vi "dashboard_motors_calibration.vi"() -> ()   [LabVIEW 2022 SP3]
panel:
  out "Applied R PWM":dbl
  in  "Tau u (s)":dbl min=0.0 max=30.0 step=0.01 format="%.2g"
  out "Applied L PWM":dbl
  in  "Stop":bool
  out "Write Count":i32
  out "Read Count":i32
  in  "Reset Communication":bool
  in  "USB Port":refnum<visa-resource-name>
  out "u":dbl format="%.2g"
  out "D":dbl format="%.2g"
  out "I":dbl format="%.2g"
  out "P":dbl format="%.2g"
  in  "Tau D (s)":dbl min=0.0 max=30.0 step=0.01 format="%.2g"
  in  "Td":dbl min=0.0 max=50.0 step=0.01 format="%.2g"
  in  "Ti":dbl=100.0 min=0.0 max=100.0 step=0.01 format="%.2g"
  in  "Kc":dbl min=0.0 max=50.0 step=0.01 format="%.2g"
  out "Flag AntiWindUp":bool
  out "Error (°)":dbl
  out "Controller":cluster{" P":dbl, "I":dbl, "D":dbl, "u":dbl}(graph)
  out "Error":cluster{" error":dbl, "Filtered_error":dbl}(graph)
  in  "PWM %":dbl(slide) min=-100.0 max=100.0 step=1.0 scale=-100.0..100.0
  in  "Setpoint (RPM)":dbl(slide) min=-1500.0 max=1500.0 step=100.0 scale=-1500.0..1500.0
  in  "Manual Control":bool=TRUE
  out "Left Motor":T1(graph)
  out "Right Motor":T2(graph)
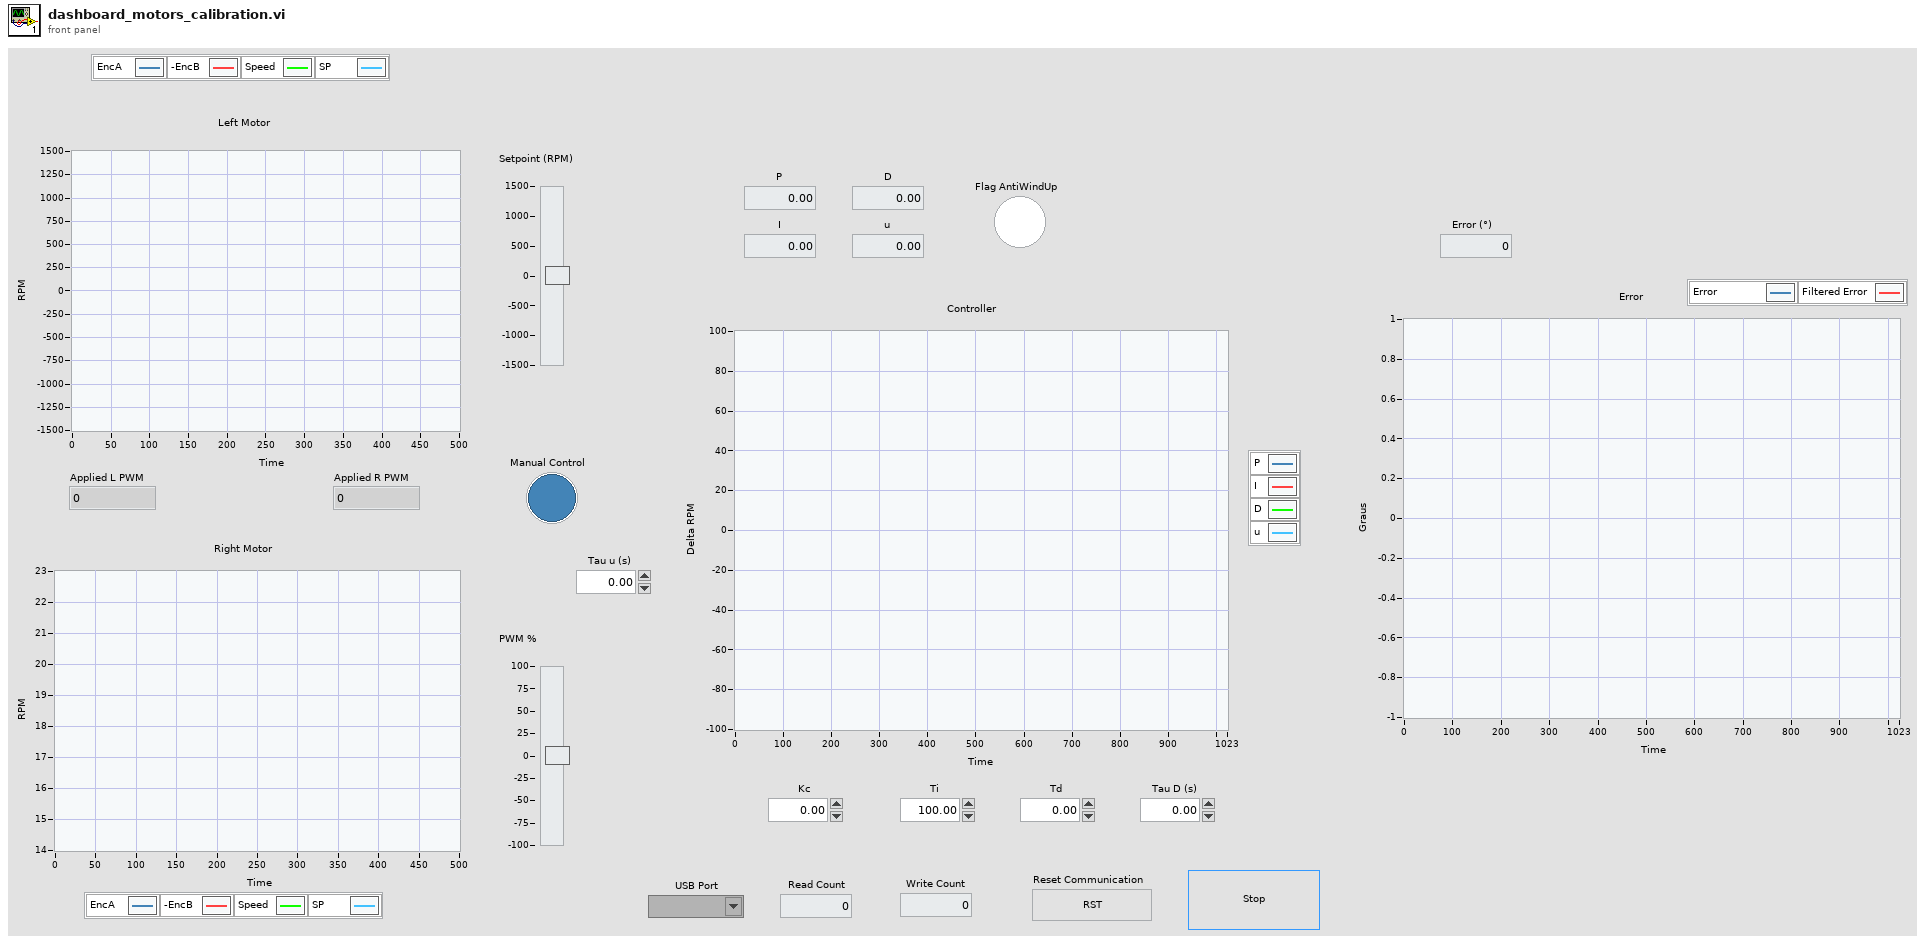
[diagram p1: front panel]
types:
  T1 = cluster{"l_sp":dbl, "l_speed":dbl, dbl, "Setpoint (RPM)":dbl}
  T2 = cluster{"r_sp":dbl, " r_speed":dbl, dbl, "Setpoint (RPM)":dbl}
  T3 = cluster{"Manual Control":bool, bool, "Setpoint (RPM)":dbl, "PWM %":dbl, "Tau u (s)":dbl, "Kc":dbl, "Ti":dbl, "Td":dbl, "Tau D (s)":dbl, dbl, dbl, dbl, dbl, dbl, dbl, dbl}
  T4 = cluster{"l_sp":dbl, "l_speed":dbl, "r_sp":dbl, " r_speed":dbl, " error":dbl, "Filtered_error":dbl, " P":dbl, "I":dbl, "D":dbl, "u":dbl, "sat_flag":bool, " IR":bool[], "A_":dbl, " B_":dbl, " C_":dbl, "D_":dbl}
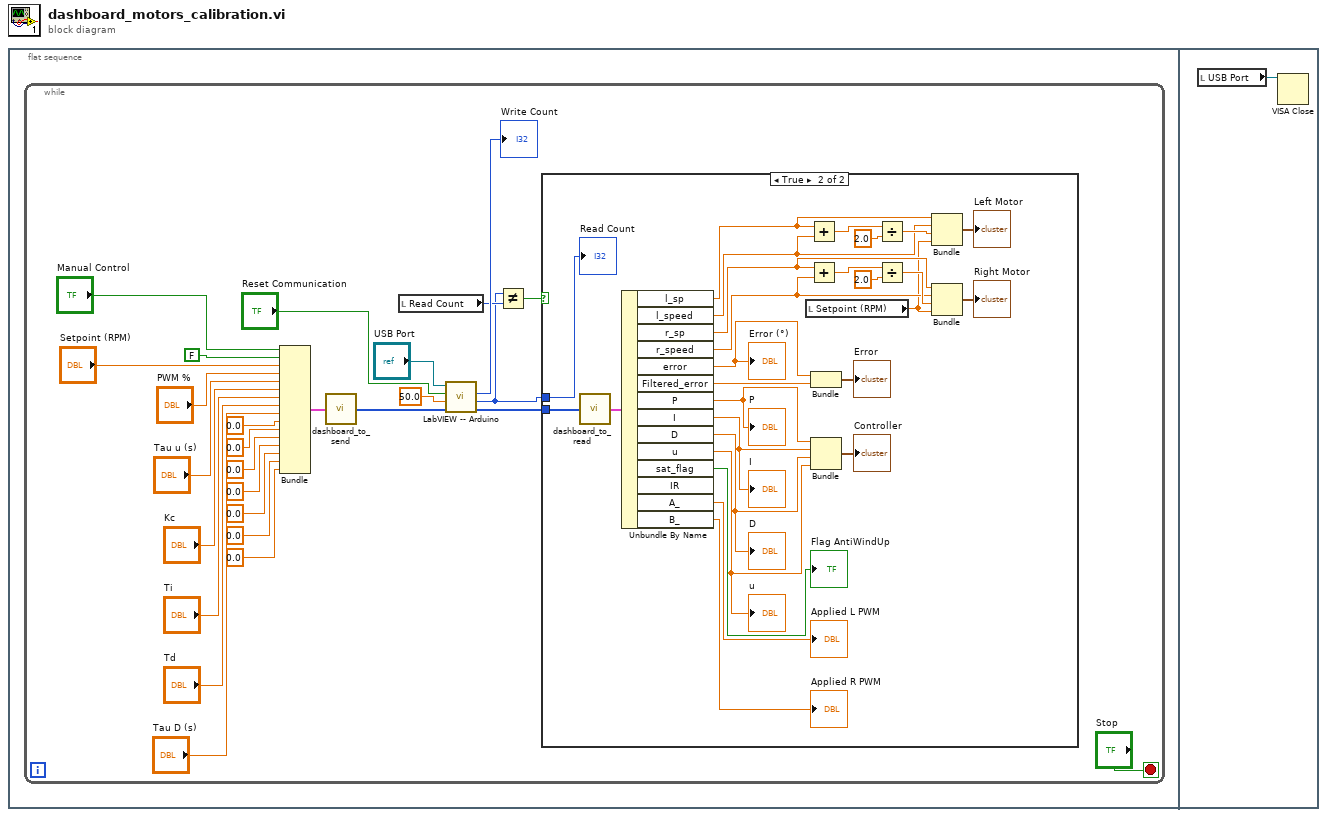
[diagram p0: block diagram]
diagram:
  n1 = flat-sequence {
    frame #0 {
      n2 = while {
        stop <- "Stop" stop-if-true
        n3 = Bundle("Manual Control"="Manual Control", FALSE, "Setpoint (RPM)"="Setpoint (RPM)", "PWM %"="PWM %", "Tau u (s)"="Tau u (s)", "Kc"="Kc", "Ti"="Ti", "Td"="Td", "Tau D (s)"="Tau D (s)", 0.0, 0.0, 0.0, 0.0, 0.0, 0.0, 0.0) -> (w9:T3)  [unwired: 1 in]
        n4 = call "dashboard_to_send.vi"("In"=w9) -> ("Output"=w8:u8[])
        n5 = local read "Read Count"() -> (w6:i32)
        n6 = call "LabVIEW -- Arduino.vi"("Data to Write"=w8, "Frequency Write"=50.0, "Reset"="Reset Communication", "VISA resource name"="USB Port") -> ("Read Data"=w4:u8[], "Read Count"=w5:i32, "Write Count"=→"Write Count":u16)  [unwired: 1 out]
        n7 = Not Equal?(x=w5, y=w6) -> (x != y?=w7:bool)
        n8 = case shown="True" w7 {
          tunnel: w5 -> [_ w54]
          tunnel: w4 -> [_ w53]
          frame False {
          }
          frame True {
            n9 = call "dashboard_to_read.vi"("In"=w53) -> ("Out"=w52:T4)
            n10 = Unbundle By Name(w52) -> ("l_sp"=w36:dbl, "l_speed"=w35:dbl, "r_sp"=w30:dbl, "r_speed"=w29:dbl, "error"=w48:dbl, "Filtered_error"=w47:dbl, "P"=w46:dbl, "I"=w45:dbl, "D"=w44:dbl, "u"=w43:dbl, "sat_flag"=→"Flag AntiWindUp":bool, "A_"=→"Applied L PWM":dbl, "B_"=→"Applied R PWM":dbl)  [unwired: 1 out]
            "Error (°)" <- w48
            "P" <- w46
            "I" <- w45
            "D" <- w44
            "u" <- w43
            n11 = local read "Setpoint (RPM)"() -> (w28:dbl)
            n12 = Add(x=w36, y=w35) -> (x+y=w38:dbl)
            n13 = Add(x=w30, y=w29) -> (x+y=w32:dbl)
            n14 = Bundle("error"=w48, "Filtered_error"=w47) -> (→"Error":cluster{" error":dbl, "Filtered_error":dbl})  [unwired: 1 in]
            n15 = Bundle("P"=w46, "I"=w45, "D"=w44, "u"=w43) -> (→"Controller":cluster{" P":dbl, "I":dbl, "D":dbl, "u":dbl})  [unwired: 1 in]
            n16 = Divide(x=w38, y=2.0) -> (x/y=w37:dbl)
            n17 = Divide(x=w32, y=2.0) -> (x/y=w31:dbl)
            n18 = Bundle("l_sp"=w36, "l_speed"=w35, w37, "Setpoint (RPM)"=w28) -> (→"Left Motor":T1)  [unwired: 1 in]
            n19 = Bundle("r_sp"=w30, "r_speed"=w29, w31, "Setpoint (RPM)"=w28) -> (→"Right Motor":T2)  [unwired: 1 in]
            "Read Count" <- w54
          }
        }
      }
    }
    frame #1 {
      n20 = local read "USB Port"() -> (w55:refnum<visa-resource-name>)
      n21 = VISA Close(VISA resource name=w55) -> ()  [unwired: 1 in, 1 out]
    }
  }
